vi "Untitled 12 (SubVI).vi"(4 "см. 1.5 in":dbl[](array[numeric]), 5 "см. 1.2 Циклов в секунду":i32(slide) scale=4.0..50.0, 6 "Кол-во выборок":i32, 7 "reference in":refnum<vi>, 9 "reference 4":refnum<vi>, 10 "reference 3":refnum<vi>, 11 "Digital in":refnum<vi>) -> (1 "Array":dbl[](array[numeric]), 2 "Модулирующий сигнал":dbl[](graph), 3 "Pulse Pattern":dbl[](array[numeric]))   [LabVIEW 2017]
uses:
  <vilib>/Analysis/NI_AALBase.lvlib
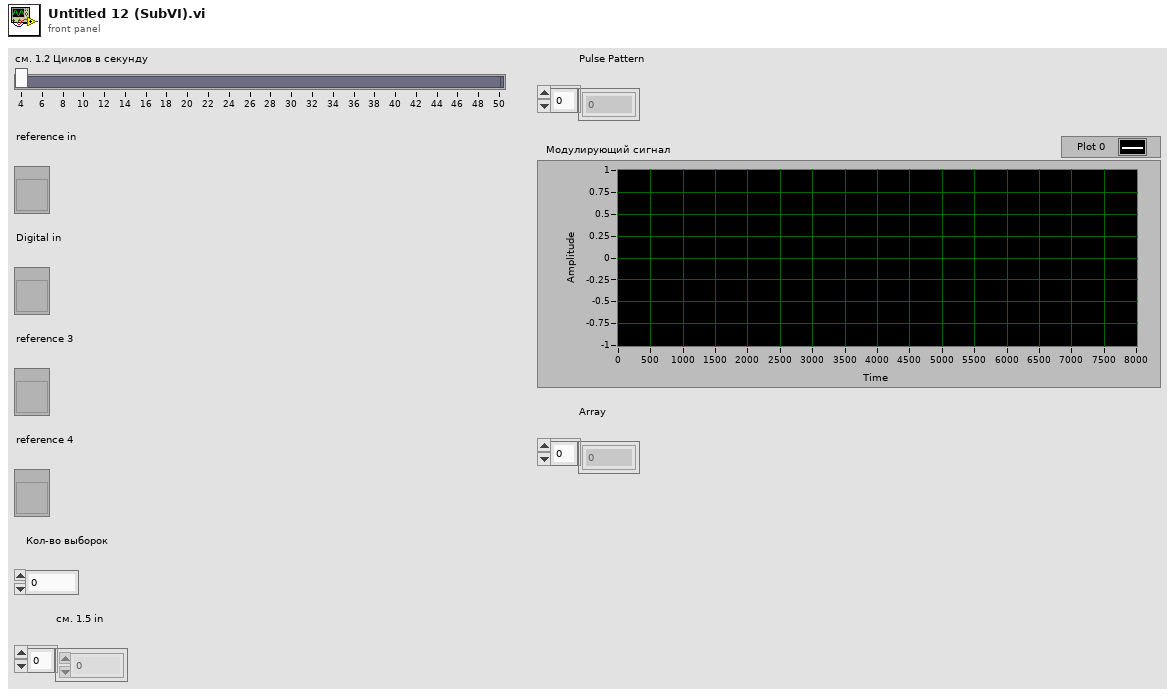
[diagram p1: front panel]
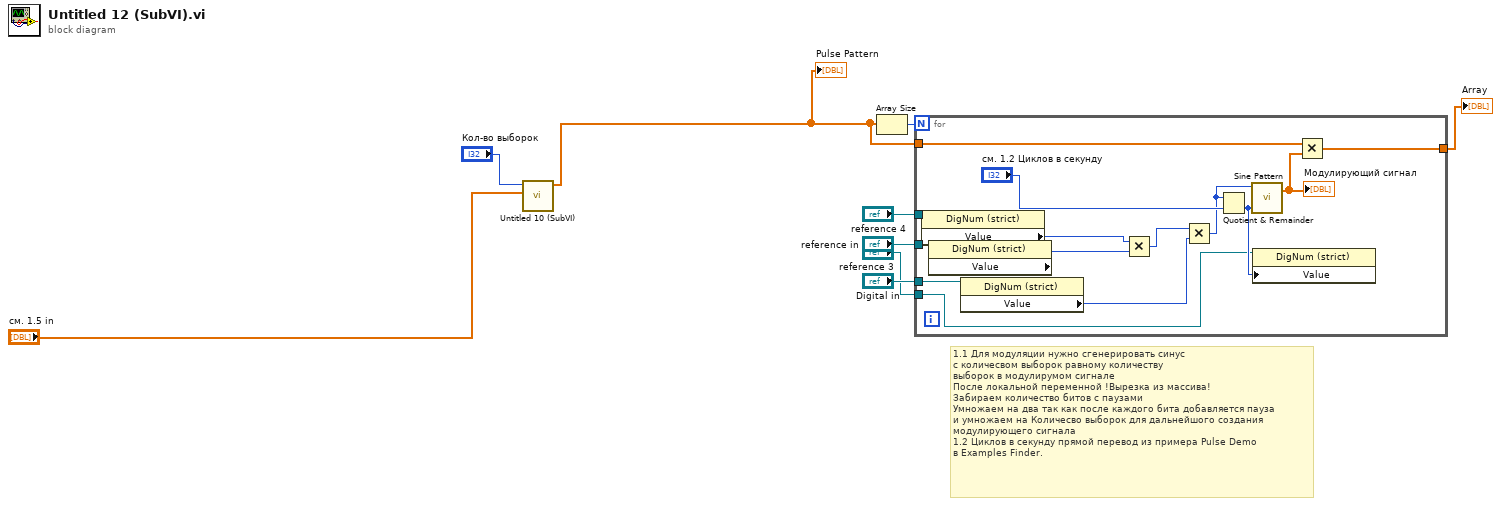
[diagram p0: block diagram]
diagram:
  # "1.1 Для модуляции нужно сгенерировать синус \nс количесвом выборок равному количеству \nвыборок в модулирумом сигнале\nПосле локальной переменной !Вырезка из массива! \nЗабираем количество битов с паузами \nУмножаем на два так как после каждого бита добавляется пауза\nи умножаем на Количесво выборок для дальнейшого создания  \nмодулирующего сигнала\n1.2 Циклов в секунду прямой перевод из примера Pulse Demo \nв Examples Finder."
  n1 = call "Untitled 10 (SubVI).vi"("см. 1.5 in"="см. 1.5 in", "Кол-во выборок"="Кол-во выборок") -> ("Pulse Pattern"=w6:dbl[])  [unwired: 9 in]
  "Pulse Pattern" <- w6
  n2 = Array Size(array=w6) -> (size(s)=w5:i32)
  n3 = for {
    N: w5 -> [_]
    tunnel: w6 -> [w22]
    tunnel: [w21] -> w7
    tunnel: "Digital in" -> [w13]
    tunnel: "reference in" -> [w12]
    tunnel: "reference 3" -> [w11]
    tunnel: "reference 4" -> [w10]
    n4 = property class="DigNum (strict)"(reference=w10) -> ("Value"=w15:i32)  [unwired: 1 in, 2 out]
    n5 = property class="DigNum (strict)"(reference=w12) -> ("Value"=w16:i32)  [unwired: 1 in, 2 out]
    n6 = property class="DigNum (strict)"(reference=w13) -> ("Value"=w19:i32)  [unwired: 1 in, 2 out]
    n7 = Multiply(x=w15, y=w16) -> (x*y=w14:i32)
    n8 = Multiply(x=w14, y=w19) -> (x*y=w18:i32)
    n9 = Quotient & Remainder(x=w18, y="см. 1.2 Циклов в секунду") -> (floor(x/y)=w17:i32)  [unwired: 1 out]
    n10 = call <vilib>:"Sine Pattern.vi"("cycles"=w17, "samples"=w18) -> ("Sinusoidal Pattern"=w20:dbl[])  [unwired: 2 in, 1 out]
    "Модулирующий сигнал" <- w20
    n11 = property class="DigNum (strict)"(reference=w11, "Value"=w17) -> ()  [unwired: 1 in, 2 out]
    n12 = Multiply(x=w22, y=w20) -> (x*y=w21:dbl[])
  }
  "Array" <- w7
